vi "Do.vi"(8 "error in (no error)":errorcluster, 10 "Actor in":refnum<class "Actor.lvclass">, 11 "Launch Server Msg in":refnum<class "Launch Server Msg.lvclass">) -> (0 "error out":errorcluster, 2 "Actor out":refnum<class "Actor.lvclass">)   [LabVIEW 2016, in "WebSocket Actors.lvlib" / "Launch Server Msg.lvclass"]
doc: "(<B>Filename</B>: Actor Framework.lvlib:Message.lvclass:Do.vi)\n\nDefines what a message does when it is received by an actor. Generally, a message instructs an actor to invoke one of its methods. By default, this method does nothing. A child class must override it to define behavior. Create a child class by using the Actor Framework Message Maker dialog box."
uses:
  Launch Server Msg.lvclass
  <vilib>/ActorFramework/Actor/Actor.lvclass
  WebSocket Server Manager/WebSocket Server Manager.lvclass
  C:/Program Files (x86)/National Instruments/LabVIEW 2016/vi.lib/ActorFramework/Actor/Actor.lvclass
  Launch Server Msg.lvclass/Launch Server Msg.ctl
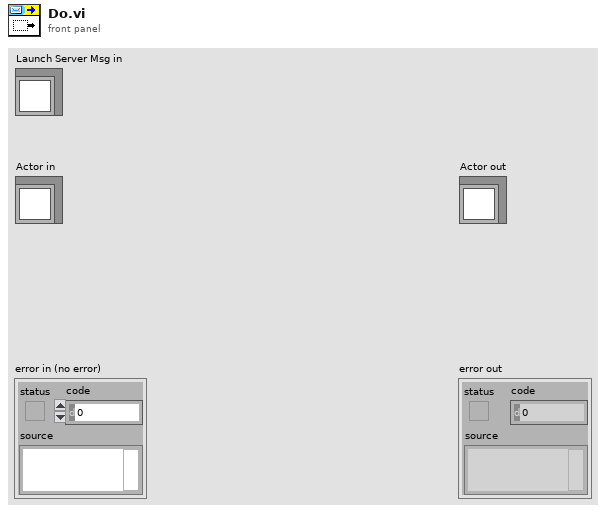
[diagram p1: front panel]
types:
  T1 = typedef "WebSocket Actors.lvlib/WebSocket Server.lvclass/Listener Settings.ctl" = cluster{"resolve remote address (T)":bool, "timeout ms (-1)":i32, "net address":u32, "port":u16}
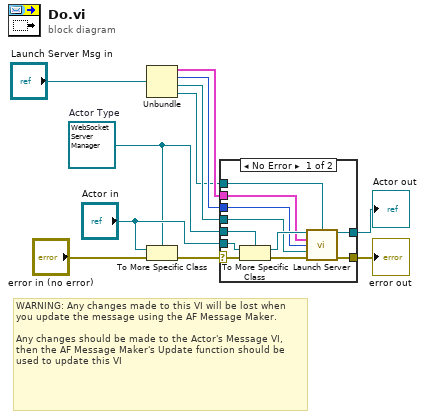
[diagram p0: block diagram]
diagram:
  w6 = refnum<class "WebSocket Server Manager.lvclass"> refnum  # Actor Type
  # "WARNING: Any changes made to this VI will be lost when you update the message using the AF Message Maker.\n\nAny changes should be made to the Actor's Message VI, then the AF Message Maker's Update function should be used to update this VI"
  n1 = Unbundle("Launch Server Msg in") -> (w5:T1, w4:i32, w3:refnum<class "Message Enqueuer.lvclass">, w2:refnum<class "WebSocket Server-Service Enqueuer Msg.lvclass">)
  n2 = To More Specific Class(target class=w6, reference="Actor in", error in="error in (no error)") -> (error out=w10:errorcluster)  [unwired: 1 out]
  n3 = case shown="No Error" w10 {
    selector: w10 -> [w22 w24]
    tunnel: [w17 w24] -> w9
    tunnel: [w16 w23] -> w8
    tunnel: "Actor in" -> [w21 w23]
    tunnel: w6 -> [w20 _]
    tunnel: w5 -> [w15 _]
    tunnel: w4 -> [w14 _]
    tunnel: w3 -> [w13 _]
    tunnel: w2 -> [w12 _]
    frame No Error {
      n4 = To More Specific Class ("Actor Cast")(target class=w20, reference=w21, error in=w22) -> (specific class reference=w19:refnum<class "WebSocket Server Manager.lvclass">, error out=w18:errorcluster)
      n5 = call "Launch Server.vi"("WebSocket Server Manager in"=w19, "Receive Server Enqueuer Handler"=w12, "Listener Settings"=w15, "Handshake timeout (5000 ms)"=w14, "Subscriber Enqueuer"=w13, "error in (no error)"=w18) -> ("WebSocket Server Manager out"=w16:refnum<class "WebSocket Server Manager.lvclass">, "error out"=w17:errorcluster)  [unwired: 8 in]
    }
    frame Error {
    }
  }
  "error out" <- w9
  "Actor out" <- w8
